vi "Set Root.vi"(8 "error in (no error)":errorcluster, 9 "Root Path":path, 11 "File Tree In":refnum<class "File Tree.lvclass">) -> (0 "error out":errorcluster, 3 "File Tree Out":refnum<class "File Tree.lvclass">)   [LabVIEW 2020, in "File Tree.lvclass"]
uses:
  File Tree.lvclass
  File Tree.lvclass/File Tree.ctl
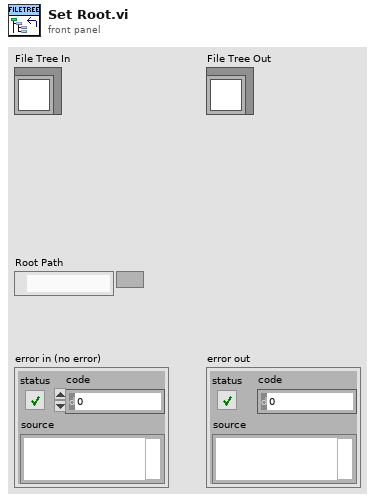
[diagram p1: front panel]
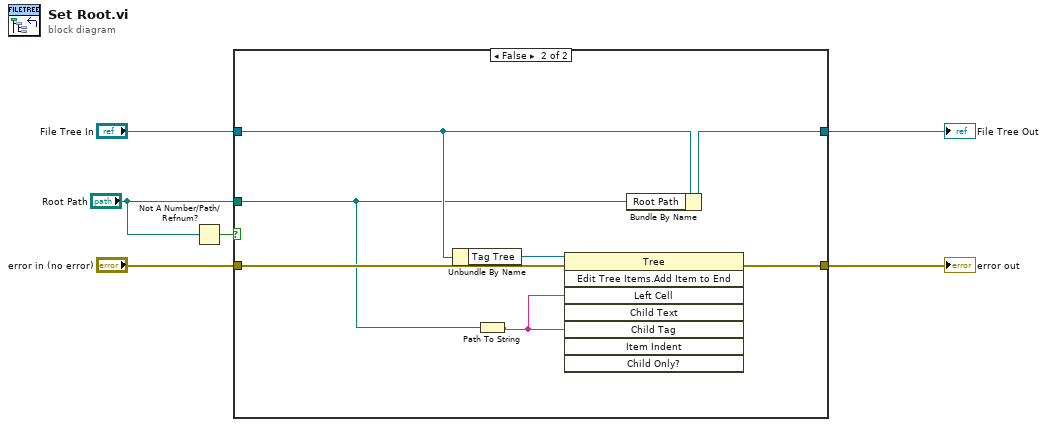
[diagram p0: block diagram]
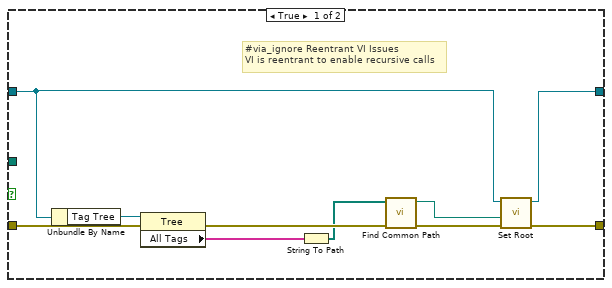
[diagram p2: hidden frame]
diagram:
  n1 = Not A Number/Path/Refnum?(number/path/refnum="Root Path") -> (NaN/Path/Refnum?=w2:bool)
  n2 = case shown="False" w2 {
    tunnel: [w13 w23] -> w6
    tunnel: "File Tree In" -> [w14 w22]
    tunnel: [w12 w21] -> w4
    tunnel: "error in (no error)" -> [w16 w20]
    tunnel: "Root Path" -> [_ w18]
    frame True {
      # "#via_ignore Reentrant VI Issues\nVI is reentrant to enable recursive calls"
      n3 = Unbundle By Name(w14) -> ("Tag Tree"=w15:refnum<vi>)
      n4 = property on="Property Node" class="Tree"(reference=w15, error in=w16) -> (error out=w11:errorcluster, "All Tags"=w10:string[])  [unwired: 1 out]
      n5 = String To Path(string=w10) -> (path=w9:path[])
      n6 = call "Find Common Path.vi"("error in (no error)"=w11, "File Paths"=w9) -> ("error out"=w7:errorcluster, "Common Path"=w8:path)  [unwired: 8 in]
      n7 = call "Set Root.vi"("error in (no error)"=w7, "Root Path"=w8, "File Tree In"=w14) -> ("error out"=w12:errorcluster, "File Tree Out"=w13:refnum<class "File Tree.lvclass">)  [unwired: 7 in]
    }
    frame False {
      n8 = Unbundle By Name(w22) -> ("Tag Tree"=w19:refnum<vi>)
      n9 = Path To String(path=w18) -> (string=w17:string)
      n10 = invoke on="Invoke Node" class="Tree" method="Edit Tree Items.Add Item to End"(reference=w19, error in=w20, "Left Cell"=w17, "Child Tag"=w17) -> (error out=w21:errorcluster)  [unwired: 4 in, 7 out]
      n11 = Bundle By Name(cluster=w22, "Root Path"=w18) -> (w23:refnum<class "File Tree.lvclass">)
    }
  }
  "File Tree Out" <- w6
  "error out" <- w4
